vi "Get State.vi"(8 "error in (no error)":errorcluster, 11 "StateMachine in":refnum<class "StateMachine.lvclass">) -> (0 "error out":errorcluster, 2 "State":string, 3 "StateMachine out":refnum<class "StateMachine.lvclass">)   [LabVIEW 2019, in "State Machine.lvlib" / "StateMachine.lvclass"]
uses:
  StateMachine.lvclass
  StateMachine.lvclass/StateMachine.ctl
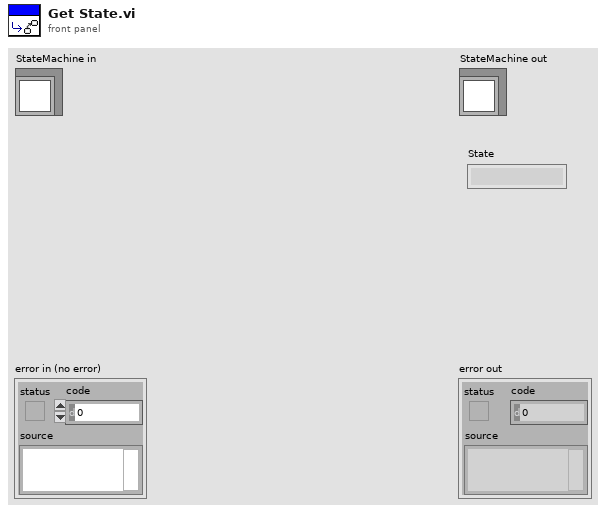
[diagram p1: front panel]
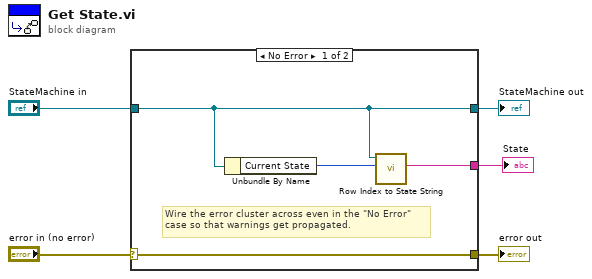
[diagram p0: block diagram]
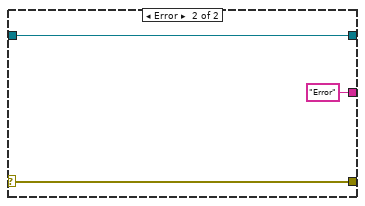
[diagram p2: hidden frame]
diagram:
  n1 = case shown="No Error" "error in (no error)" {
    selector: "error in (no error)" -> [w9 w12]
    tunnel: [w9 w12] -> w4
    tunnel: [w7 w11] -> w2
    tunnel: "StateMachine in" -> [w7 w11]
    tunnel: [w6 "Error" ("State String")] -> w1
    frame No Error {
      # "Wire the error cluster across even in the \"No Error\"\ncase so that warnings get propagated."
      n2 = Unbundle By Name(w7) -> ("Current State"=w8:i32)
      n3 = call-dynamic "Row Index to State String.vi"("Row Index"=w8, "StateMachine in"=w7) -> ("State String"=w6:string)  [unwired: 7 in, 2 out]
    }
    frame Error {
    }
  }
  "error out" <- w4
  "StateMachine out" <- w2
  "State" <- w1
